vi "Launch_Pre_Loop_Initialization_FGV.vi"(8 "error in (no error)":errorcluster, 11 "VI in":refnum<vi>) -> (0 "error out":errorcluster, 3 "User Event out":refnum<user-event>)   [LabVIEW 2024, in "LaunchTest.lvlib"]
doc: "This VI\n------------------------------------------------\nPer_Loop_Initialize\n------------------------------------------------\n-Generate the Communication Queue Reference with FGV.\n-Get the Common User Events Reference at Application Level."
uses:
  LaunchTest.lvlib
  PrivateControls/Launch_FGV_Queue_Control.ctl
  support/Message Queue/Launch_Message Cluster.ctl
  support/Message Queue/Launch_Message Queue.lvlib
  UserEvents/Controls/User_Events_Action_Control.ctl
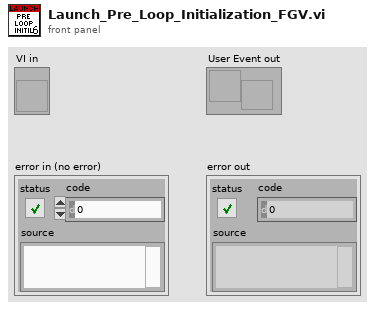
[diagram p1: front panel]
types:
  T1 = typedef "LaunchTest.lvlib/User_Events_Action_Control.ctl" = enum16{"Get", "Create", "Destroy"}
  T2 = typedef "LaunchTest.lvlib/Launch_Message Queue.lvlib/Launch_Message Cluster.ctl" = cluster{"Message":string, "Message Data":variant}
  T3 = typedef "LaunchTest.lvlib/Launch_FGV_Queue_Control.ctl" = enum16{"Release", "Get", "Set", "Flush"}
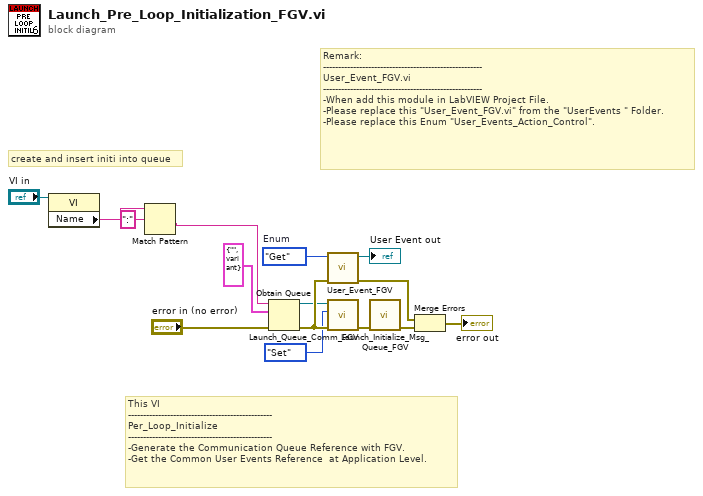
[diagram p0: block diagram]
diagram:
  w10 = User_Events_Action_Control."Get"  # Enum
  # "Remark:\n-----------------------------------------------------\nUser_Event_FGV.vi\n-----------------------------------------------------\n-When add this module in LabVIEW Project File.\n-Please replace this \"User_Event_FGV.vi\" from the \"UserEvents \" Folder.\n-Please replace this Enum \"User_Events_Action_Control\"."
  # "This VI\n------------------------------------------------\nPer_Loop_Initialize\n------------------------------------------------\n-Generate the Communication Queue Reference with FGV.\n-Get the Common User Events Reference  at Application Level."
  # "create and insert initi into queue"
  n1 = property class="VI"(reference="VI in") -> ("Name"=w3:string)  [unwired: 1 in, 2 out]
  n2 = Match Pattern(string=w3, regular expression=":") -> (after substring=w2:string)  [unwired: 1 in, 3 out]
  n3 = Obtain Queue(name (unnamed)=w2, element data type=T2 {"Message"="", "Message Data"=variant} ("Message Cluster"), error in (no error)="error in (no error)") -> (queue out=w9:refnum<queue>, error out=w11:errorcluster)  [unwired: 2 in, 1 out]
  n4 = call "User_Event_FGV.vi"("error in (no error)"=w11, "Enum"=w10) -> ("error out"=w13:errorcluster, "User Event out"=→"User Event out":refnum<user-event>)  [unwired: 8 in]
  n5 = call "Launch_Queue_Comm_FGV.vi"("error in (no error)"=w11, "Enum"=Launch_FGV_Queue_Control."Set", "queue in"=w9) -> ("error Out"=w7:errorcluster)  [unwired: 7 in, 1 out]
  n6 = call "Launch_Initialize_Msg_Queue_FGV.vi"("error in (no error)"=w7) -> ("error out"=w14:errorcluster)  [unwired: 10 in]
  n7 = Merge Errors(w13, w14) -> (→"error out":errorcluster)
